vi "LogView.vi"(2 "error in":errorcluster caption="错误输入（无错误）", 3 "StrIn":string) -> (0 "error out":errorcluster caption="错误输出", 1 "StrOut":string)   [LabVIEW 2013]
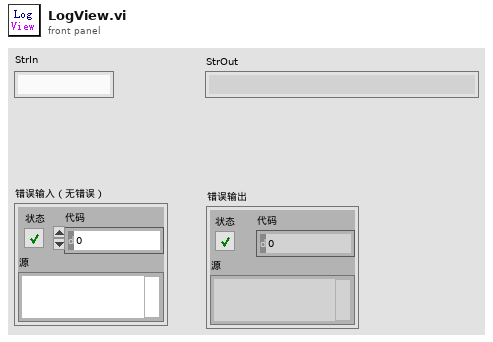
[diagram p1: front panel]
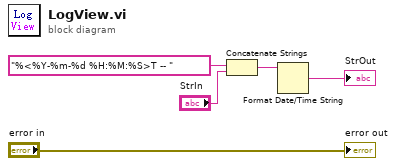
[diagram p0: block diagram]
diagram:
  n1 = Concatenate Strings("%<%Y-%m-%d %H:%M:%S>T -- " ("时间格式字符串(%c)"), "StrIn") -> (w2:string)
  n2 = Format Date/Time String(time format string (%c)=w2) -> (date/time string=→"StrOut":string)  [unwired: 2 in]
  "error out" <- "error in"
